vi "Start Sequence Acquisition.vi"(8 "error in (no error)":errorcluster, 11 "Stage in":refnum<class "Stage.lvclass">) -> (0 "error out":errorcluster, 3 "Stage out":refnum<class "Stage.lvclass">)   [LabVIEW 2020, in "Stage.lvlib" / "Stage.lvclass"]
uses:
  Stage.lvclass
  C:/Program Files/National Instruments/LabVIEW 2020/vi.lib/ActorFramework/Actor/Actor.lvclass
  Stage.lvclass/Stage.ctl
  <vilib>/ActorFramework/Actor/Actor.lvclass/Actor.ctl
  <vilib>/ActorFramework/Message Enqueuer/Message Enqueuer.lvclass/Message Enqueuer.ctl
  <vilib>/ActorFramework/Message Enqueuer/Init from Existing Queue.vi
  <vilib>/ActorFramework/Message Enqueuer/Enqueue.vi
  Stage Messages/Start Sequence Acquisition Msg/Start Sequence Acquisition Msg.lvclass
  C:/Program Files/National Instruments/LabVIEW 2020/vi.lib/ActorFramework/Message/Message.lvclass
  <vilib>/ActorFramework/Message Priority Queue/Priority Enqueue.vi
  <vilib>/ActorFramework/Message Enqueuer/Message Enqueuer.lvclass
  <vilib>/ActorFramework/Actor/Actor.lvclass
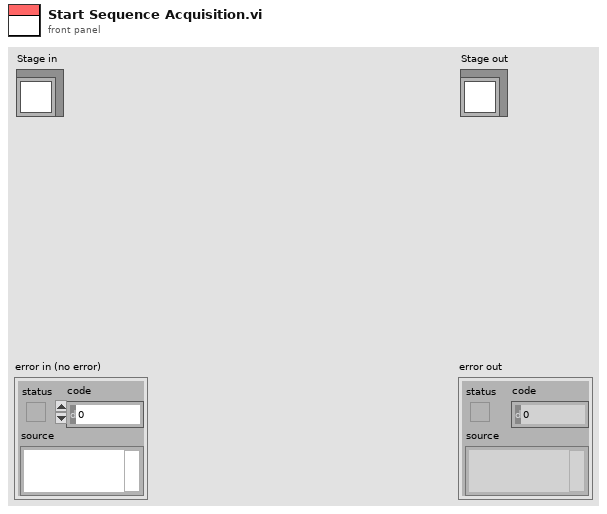
[diagram p1: front panel]
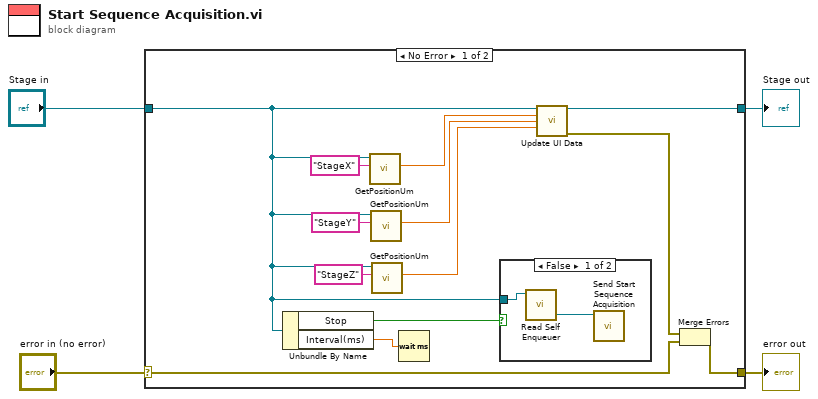
[diagram p0: block diagram]
diagram:
  n1 = case shown="No Error" "error in (no error)" {
    selector: "error in (no error)" -> [w8 w21]
    tunnel: [w16 w21] -> w3
    tunnel: [w17 w20] -> w1
    tunnel: "Stage in" -> [w5 w20]
    frame No Error {
      n2 = Unbundle By Name(w5) -> ("Stop"=w7:bool, "Interval(ms)"=w6:dbl)
      n3 = call-dynamic "GetPositionUm.vi"("Stage Label"="StageX", "Stage in"=w5) -> ("Stage Position"=w11:dbl)  [unwired: 7 in, 2 out]
      n4 = call-dynamic "GetPositionUm.vi"("Stage Label"="StageY", "Stage in"=w5) -> ("Stage Position"=w10:dbl)  [unwired: 7 in, 2 out]
      n5 = call-dynamic "GetPositionUm.vi"("Stage Label"="StageZ", "Stage in"=w5) -> ("Stage Position"=w9:dbl)  [unwired: 7 in, 2 out]
      n6 = Wait (ms)(milliseconds to wait=w6) -> ()  [unwired: 1 out]
      n7 = case shown="False" w7 {
        tunnel: w5 -> [w19 _]
        frame False {
          n8 = call <vilib>:"Read Self Enqueuer.vi"("Actor"=w19) -> ("Self Enqueuer"=w18:refnum<class "Message Enqueuer.lvclass">)  [unwired: 10 in]
          n9 = call "Send Start Sequence Acquisition.vi"("Message Enqueuer"=w18) -> ()  [unwired: 9 in, 2 out]
        }
        frame True {
        }
      }
      n10 = call-dynamic "Update UI Data.vi"("Stage in"=w5, "Stage X Position"=w11, "Stage Y Position"=w10, "Stage Z Position"=w9) -> ("Stage out"=w17:refnum<class "Stage.lvclass">, "error out"=w15:errorcluster)  [unwired: 10 in]
      n11 = Merge Errors(w15, w8) -> (w16:errorcluster)
    }
    frame Error {
    }
  }
  "error out" <- w3
  "Stage out" <- w1
